vi "Copy Messenger Reference.vi"(8 "error in (no error)":errorcluster, 9 "Child In":refnum<class "System Actor.lvclass">, 11 "System Actor in":refnum<class "System Actor.lvclass">) -> (0 "error out":errorcluster, 3 "Child out":refnum<class "System Actor.lvclass">)   [LabVIEW 2024, in "System Actor.lvclass"]
uses:
  System Actor.lvclass
  System Actor.lvclass/System Actor.ctl
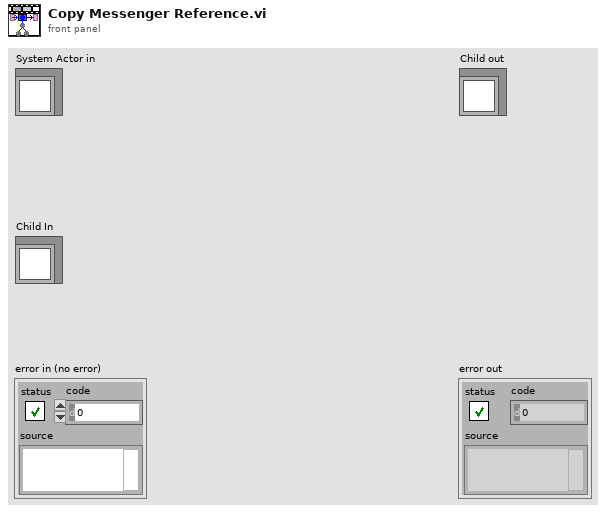
[diagram p1: front panel]
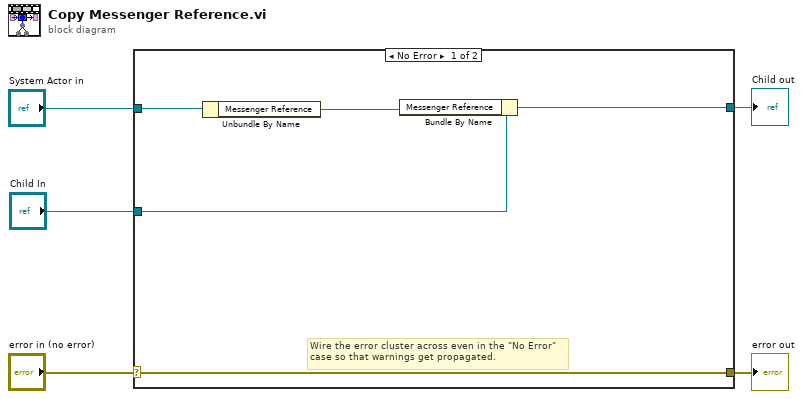
[diagram p0: block diagram]
diagram:
  n1 = case shown="No Error" "error in (no error)" {
    selector: "error in (no error)" -> [w10 w12]
    tunnel: [w10 w12] -> w4
    tunnel: [w8 w11] -> w2
    tunnel: "System Actor in" -> [w7 _]
    tunnel: "Child In" -> [w9 w11]
    frame No Error {
      # "Wire the error cluster across even in the \"No Error\"\ncase so that warnings get propagated."
      n2 = Unbundle By Name(w7) -> ("Messenger Reference"=w6:refnum<data-value>)
      n3 = Bundle By Name(cluster=w9, "Messenger Reference"=w6) -> (w8:refnum<class "System Actor.lvclass">)
    }
    frame Error {
    }
  }
  "error out" <- w4
  "Child out" <- w2
